vi "Request Stop.vi"(8 "error in (no error)":errorcluster, 9 "Critical (F)":bool, 11 "module in":refnum<class "UIManager.lvclass">) -> (0 "error out":errorcluster, 3 "module out":refnum<class "UIManager.lvclass">)   [LabVIEW 2024, in "UIManager.lvclass"]
uses:
  UIManager.lvclass
  UIManager.lvclass/UIManager.ctl
  C:/Git/JA/JQMH/RQMHCore/ModuleCore/Module.lvclass
  C:/Git/JA/JQMH/ModuleTemplates/UIManager/UIManager.lvclass
  RQMHCore/ModuleCore/Module.lvclass
  Request Stop.ctl
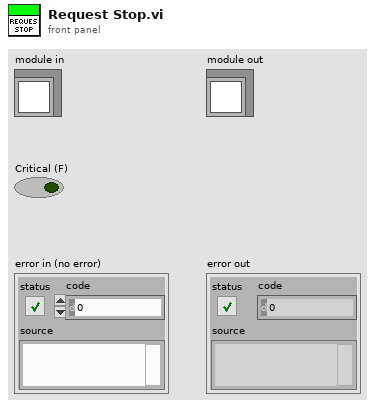
[diagram p1: front panel]
types:
  T1 = typedef "UIManager.lvclass/Request Stop.ctl" = cluster{"Module":refnum<class "Module.lvclass">, "Critical":bool}
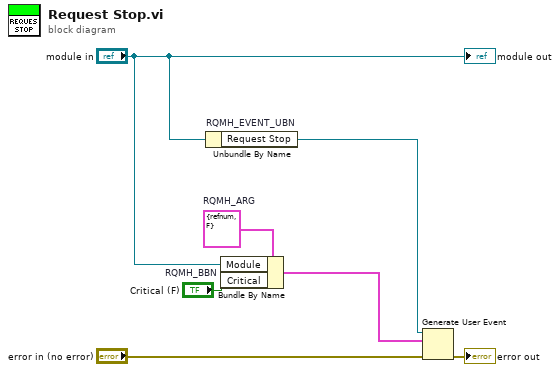
[diagram p0: block diagram]
diagram:
  w4 = T1 {"Module"=refnum, "Critical"=FALSE}  # RQMH_ARG
  n1 = Unbundle By Name "RQMH_EVENT_UBN"("module in") -> ("Request Stop"=w7:refnum<user-event>)
  n2 = Bundle By Name "RQMH_BBN"(cluster=w4, "Module"="module in", "Critical"="Critical (F)") -> (w3:T1)
  n3 = Generate User Event(user event=w7, event data cluster=w3, error in="error in (no error)") -> (error out=→"error out":errorcluster)  [unwired: 1 in, 1 out]
  "module out" <- "module in"
